vi "BinaryThreshold.vi"(2 "threshold":cluster{u8, u8}(slide)={0, 44} scale=0.0..255.0, 3 "Image In":T1 {"Dialogs" format="%.0b"}) -> (1 "Image Out":T1 {"Dialogs" format="%.0b"})   [LabVIEW 2024]
doc: "This VI takes as an input a threshold (a cluster containing the upper and lower bounds) and an 8 bit input image. It then creates a binary image based upon the upper and lower bounds of the threshold. For instance, pixels with a value between the threshold bounds will be a one. All others will be a zero.\n\nIf the input image is RGB (24 bit), the threshold will be applied to the 8 bit grayscale representation of the input image."
uses:
  <userlib>/ImageProcessing/QTLIB_2595_LV86/QT_Image.ctl
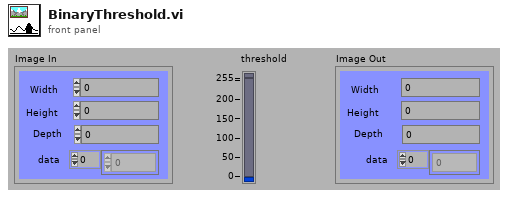
[diagram p1: front panel]
types:
  T1 = typedef "QT_Image.ctl" = cluster{"Width":i32, "Height":i32, "Depth":i32, "data":u8[], "Compressed data":u8[], "Color table":u32[], "Duration":i32, "Options":i32, "Timestamp":i32, "ID":i32, "Reserved":i32, "Dialogs":u32}
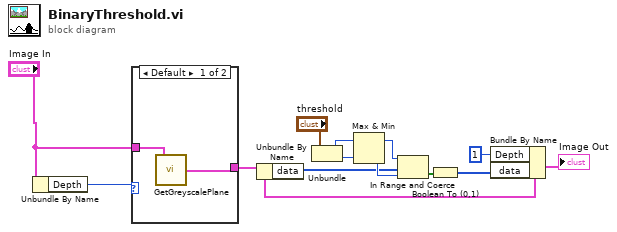
[diagram p0: block diagram]
diagram:
  n1 = Unbundle By Name("Image In") -> ("Depth"=w12:i32)
  n2 = case shown="Default" w12 {
    tunnel: "Image In" -> [w15 w16]
    tunnel: [w14 w16] -> w2
    frame Default {
      n3 = call <userlib>:"GetGreyscalePlane.vi"("Image In"=w15) -> ("Greyscale  Out"=w14:T1)
    }
    frame 1, 8 {
    }
  }
  n4 = Unbundle By Name(w2) -> ("data"=w6:u8[])
  n5 = Unbundle("threshold") -> (w3:u8, w4:u8)
  n6 = Max & Min(x=w3, y=w4) -> (max(x,y)=w5:u8, min(x,y)=w8:u8)
  n7 = In Range and Coerce(upper limit=w5, x=w6, lower limit=w8) -> (In Range?=w7:bool[])  [unwired: 1 out]
  n8 = Boolean To (0,1)(Boolean=w7) -> (0, 1=w10:i16[])
  n9 = Bundle By Name(cluster=w2, "Depth"=1, "data"=w10) -> (→"Image Out":T1)
